vi "oa_CIC Filter Length.vi"(7 "CIC filter settings":T1={"interpolation/decimation factor"=2, "stages"=2, "lag"=1}) -> (8 "CIC filter length":i32)   [LabVIEW 2017, in "SoundVib_Resampling.lvlib"]
uses:
  <vilib>/addons/Sound and Vibration/Order Analysis/Resample Order Tracking/SoundVib_Resampling.lvlib
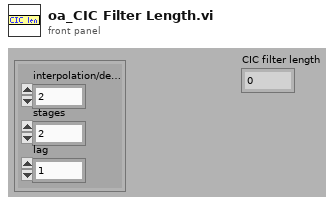
[diagram p1: front panel]
types:
  T1 = cluster{"interpolation/decimation factor":i32, "stages":i32, "lag":i32}
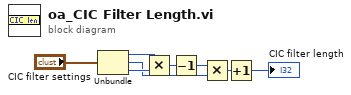
[diagram p0: block diagram]
diagram:
  n1 = Unbundle("CIC filter settings") -> ("interpolation/decimation factor"=w5:i32, "stages"=w3:i32, "lag"=w4:i32)
  n2 = Multiply(x=w5, y=w4) -> (x*y=w8:i32)
  n3 = Decrement(x=w8) -> (x-1=w7:i32)
  n4 = Multiply(x=w7, y=w3) -> (x*y=w6:i32)
  n5 = Increment(x=w6) -> (x+1=→"CIC filter length":i32)
